vi "Automatic CE-CERT Inverter MODBUS TCP-IP Power Factor.vi"() -> ()   [LabVIEW 2018]
uses:
  <vilib>/Plasmionique/MB Master/MB_Master_TCP/MB_Master_TCP.lvclass
  C:/Program Files (x86)/National Instruments/LabVIEW 2018/vi.lib/Plasmionique/MB Master/MB_Master/MB_Master.lvclass
  <vilib>/Plasmionique/MB Master/MB Master.lvlib
panel:
  in  "Number of iterations":i32
  in  "Seconds to wait before commands sent":u32
  in  "power factor set point":u16
  out "Power Factor Format Error (0)":u16
  out "3035 Register Value":u16
  out "Power Factor Mode Read Back (Step 10)":u16
  out "Power Factor Operation Error (Step 9)(Can Read 0 or 10)":u16
  out "Power Factor Operation Error (Step 1)(Should Read 0)":u16
  in  "IP Address":string
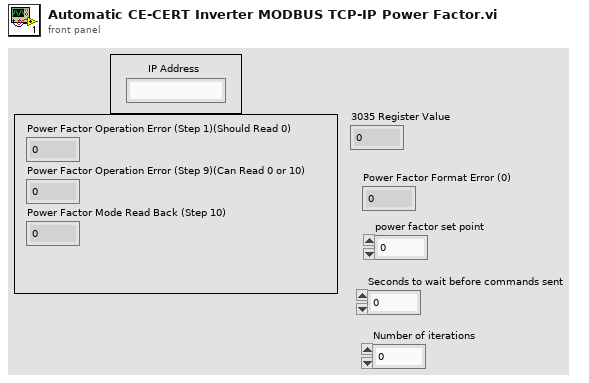
[diagram p1: front panel]
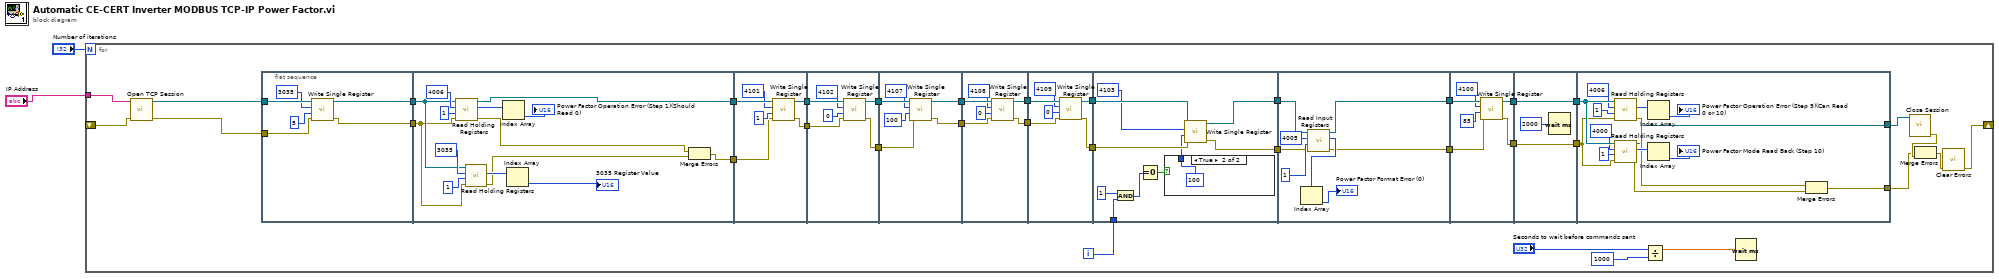
[diagram p0: block diagram]
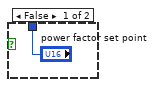
[diagram p2: hidden frame]
diagram:
  n1 = for {
    N: "Number of iterations" -> [_]
    tunnel: "IP Address" -> [w33]
    shift-right: [w25] -> _
    shift-left: _ -> [w31]
    i -> [w3]
    n2 = call <vilib>:"Open TCP Session.vi"("error in (no error)"=w31, "IP Address"=w33) -> ("error out"=w30:errorcluster, "MB_TCP session"=w32:refnum<class "MB_Master_TCP.lvclass">)  [unwired: 8 in]
    n3 = flat-sequence {
      tunnel: w32 -> [w43]
      tunnel: [w40] -> w24
      tunnel: w30 -> [w39]
      tunnel: [w38] -> w23
      tunnel: [w55] -> w22
      tunnel: w24 -> [w50]
      tunnel: w23 -> [w47]
      tunnel: [w44] -> w21
      tunnel: w22 -> [w63]
      tunnel: [w60] -> w20
      tunnel: w21 -> [w59]
      tunnel: [w58] -> w19
      tunnel: w20 -> [w69]
      tunnel: [w66] -> w18
      tunnel: w19 -> [w65]
      tunnel: [w64] -> w17
      tunnel: w18 -> [w75]
      tunnel: [w74] -> w16
      tunnel: w17 -> [w71]
      tunnel: [w70] -> w15
      tunnel: w16 -> [w81]
      tunnel: [w78] -> w14
      tunnel: w15 -> [w77]
      tunnel: [w76] -> w13
      tunnel: w14 -> [w87]
      tunnel: [w84] -> w12
      tunnel: w13 -> [w83]
      tunnel: [w82] -> w11
      tunnel: w12 -> [w97]
      tunnel: [w95] -> w37
      tunnel: w11 -> [w94]
      tunnel: [w93] -> w29
      tunnel: w3 -> [w91]
      tunnel: w37 -> [w107]
      tunnel: [w106] -> w36
      tunnel: w29 -> [w101]
      tunnel: [w100] -> w28
      tunnel: w36 -> [w113]
      tunnel: [w110] -> w35
      tunnel: w28 -> [w109]
      tunnel: [w108] -> w26
      tunnel: w35 -> [w116]
      tunnel: [w116] -> w34
      tunnel: [w114] -> w27
      tunnel: w26 -> [w114]
      tunnel: w34 -> [w130]
      tunnel: w27 -> [w121]
      tunnel: [w118] -> w5
      tunnel: [w117] -> w7
      frame #0 {
        n4 = call <vilib>:"Write Single Register.vi"("error in (no error)"=w39, "value"=u16 5, "address"=u16 3035, "MB session in"=w43) -> ("error out"=w38:errorcluster, "MB session out"=w40:refnum<class "MB_Master_TCP.lvclass">)  [unwired: 6 in]
      }
      frame #1 {
        n5 = call <vilib>:"Read Holding Registers.vi"("error in (no error)"=w47, "quantity"=u16 1, "starting address"=u16 4006, "MB session in"=w50) -> ("error out"=w46:errorcluster, "Registers"=w57:u16[], "MB session out"=w55:refnum<class "MB_Master_TCP.lvclass">)  [unwired: 5 in]
        n6 = call <vilib>:"Read Holding Registers.vi"("error in (no error)"=w47, "quantity"=u16 1, "starting address"=u16 3035, "MB session in"=w50) -> ("error out"=w45:errorcluster, "Registers"=w49:u16[])  [unwired: 5 in, 1 out]
        n7 = Index Array(array=w57) -> (element=→"Power Factor Operation Error (Step 1)(Should Read 0)":u16)  [unwired: 1 in]
        n8 = Index Array(array=w49) -> (element=→"3035 Register Value":u16)  [unwired: 1 in]
        n9 = Merge Errors(w46, w45) -> (w44:errorcluster)
      }
      frame #2 {
        n10 = call <vilib>:"Write Single Register.vi"("error in (no error)"=w59, "value"=u16 1, "address"=u16 4101, "MB session in"=w63) -> ("error out"=w58:errorcluster, "MB session out"=w60:refnum<class "MB_Master_TCP.lvclass">)  [unwired: 6 in]
      }
      frame #3 {
        n11 = call <vilib>:"Write Single Register.vi"("error in (no error)"=w65, "value"=u16 0, "address"=u16 4102, "MB session in"=w69) -> ("error out"=w64:errorcluster, "MB session out"=w66:refnum<class "MB_Master_TCP.lvclass">)  [unwired: 6 in]
      }
      frame #4 {
        n12 = call <vilib>:"Write Single Register.vi"("error in (no error)"=w71, "value"=u16 100, "address"=u16 4107, "MB session in"=w75) -> ("error out"=w70:errorcluster, "MB session out"=w74:refnum<class "MB_Master_TCP.lvclass">)  [unwired: 6 in]
      }
      frame #5 {
        n13 = call <vilib>:"Write Single Register.vi"("error in (no error)"=w77, "value"=u16 0, "address"=u16 4108, "MB session in"=w81) -> ("error out"=w76:errorcluster, "MB session out"=w78:refnum<class "MB_Master_TCP.lvclass">)  [unwired: 6 in]
      }
      frame #6 {
        n14 = call <vilib>:"Write Single Register.vi"("error in (no error)"=w83, "value"=u16 0, "address"=u16 4109, "MB session in"=w87) -> ("error out"=w82:errorcluster, "MB session out"=w84:refnum<class "MB_Master_TCP.lvclass">)  [unwired: 6 in]
      }
      frame #7 {
        n15 = And(x=1, y=w91) -> (x .and. y?=w88:i32)
        n16 = Equal To 0?(x=w88) -> (x = 0?=w89:bool)
        n17 = case shown="True" w89 {
          tunnel: ["power factor set point" u16 100 ("power factor set point")] -> w92
          frame False {
          }
          frame True {
          }
        }
        n18 = call <vilib>:"Write Single Register.vi"("error in (no error)"=w94, "value"=w92, "address"=u16 4103, "MB session in"=w97) -> ("error out"=w93:errorcluster, "MB session out"=w95:refnum<class "MB_Master_TCP.lvclass">)  [unwired: 6 in]
      }
      frame #8 {
        n19 = call <vilib>:"Read Input Registers.vi"("error in (no error)"=w101, "quantity"=u16 1, "starting address"=u16 4005, "MB session in"=w107) -> ("error out"=w100:errorcluster, "Registers"=w103:u16[], "MB session out"=w106:refnum<class "MB_Master_TCP.lvclass">)  [unwired: 5 in]
        n20 = Index Array(array=w103) -> (element=→"Power Factor Format Error (0)":u16)  [unwired: 1 in]
      }
      frame #9 {
        n21 = call <vilib>:"Write Single Register.vi"("error in (no error)"=w109, "value"=u16 85, "address"=u16 4100, "MB session in"=w113) -> ("error out"=w108:errorcluster, "MB session out"=w110:refnum<class "MB_Master_TCP.lvclass">)  [unwired: 6 in]
      }
      frame #10 {
        n22 = Wait (ms)(milliseconds to wait=u32 2000) -> ()  [unwired: 1 out]
      }
      frame #11 {
        n23 = call <vilib>:"Read Holding Registers.vi"("error in (no error)"=w121, "quantity"=u16 1, "starting address"=u16 4006, "MB session in"=w130) -> ("error out"=w120:errorcluster, "Registers"=w125:u16[])  [unwired: 5 in, 1 out]
        n24 = call <vilib>:"Read Holding Registers.vi"("error in (no error)"=w121, "quantity"=u16 1, "starting address"=u16 4000, "MB session in"=w130) -> ("error out"=w119:errorcluster, "Registers"=w124:u16[], "MB session out"=w117:refnum<class "MB_Master_TCP.lvclass">)  [unwired: 5 in]
        n25 = Index Array(array=w125) -> (element=→"Power Factor Operation Error (Step 9)(Can Read 0 or 10)":u16)  [unwired: 1 in]
        n26 = Index Array(array=w124) -> (element=→"Power Factor Mode Read Back (Step 10)":u16)  [unwired: 1 in]
        n27 = Merge Errors(w120, w119) -> (w118:errorcluster)
      }
    }
    n28 = Divide(x="Seconds to wait before commands sent", y=u32 1000) -> (x/y=w9:dbl)
    n29 = Wait (ms)(milliseconds to wait=w9) -> ()  [unwired: 1 out]
    n30 = call-dynamic "Close Session.vi"("MB TCP session"=w7) -> ("error out"=w6:errorcluster)  [unwired: 10 in]
    n31 = Merge Errors(w5, w6) -> (w4:errorcluster)
    n32 = call <vilib>:"Clear Errors.vi"("error in (no error)"=w4) -> ("error out"=w25:errorcluster)  [unwired: 5 in, 1 out]
  }
